vi "DrivePath-C.vi"(11 "Params":string[][](array[string])) -> ()   [LabVIEW 2017]
uses:
  C:/Users/Bendethic/Desktop/AutoRoutineCreator/RoutineData.vi
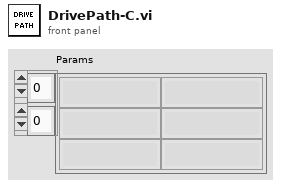
[diagram p1: front panel]
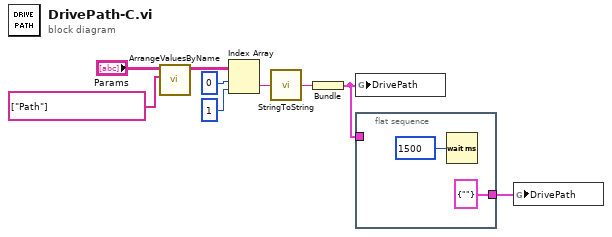
[diagram p0: block diagram]
diagram:
  n1 = call "ArrangeValuesByName.vi"("Names"=string[] ["Path"], "Names/Values in"="Params") -> ("Names/Values Out"=w5:string[][])  [unwired: 9 in]
  n2 = Index Array(array=w5, index (row)=0, index (col)=1) -> (element=w1:string)
  n3 = call "StringToString.vi"("String"=w1) -> ("Output"=w8:string)
  n4 = Bundle("Output"=w8) -> (w9:cluster{"Output":string})  [unwired: 1 in]
  n5 = global write "RoutineData.vi" "DrivePath"(w9) -> ()
  n6 = flat-sequence {
    tunnel: w9 -> [_]
    tunnel: [cluster{"Path":string} {"Path"=""} ("DrivePath")] -> w7
    frame #0 {
      n7 = Wait (ms)(milliseconds to wait=u32 1500) -> ()  [unwired: 1 out]
    }
  }
  n8 = global write "RoutineData.vi" "DrivePath"(w7) -> ()
